vi "Close.vi"(8 "error in (no error)":errorcluster, 11 "IVI_Class in":refnum<class "IVI_Class.lvclass">) -> (0 "error out":errorcluster, 3 "IVI_Class out":refnum<class "IVI_Class.lvclass">)   [LabVIEW 2018, in "ScopePlugins.lvlib" / "IVI_Class.lvclass"]
doc: "Closes the session to the instrument."
uses:
  IVI_Class.lvclass
  C:/projects/ICDAS/NistPluggableModules/Scope/ScopePlugins/ScopePluginBaseClass/ScopePluginsBase.lvclass
  ScopePluginBaseClass/ScopePluginsBase.lvclass/ScopePluginsBase.ctl
  ScopePluginBaseClass/Accessors/Read Channels.vi
  ScopePluginBaseClass/Accessors/Write Channels.vi
  ScopePluginBaseClass/ScopePluginsBase.lvclass
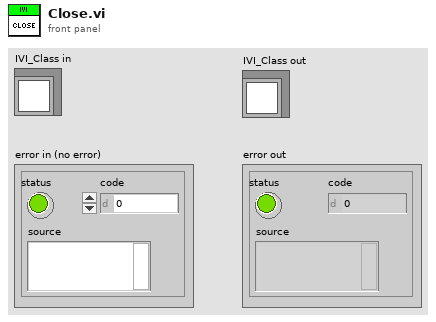
[diagram p1: front panel]
types:
  T1 = typedef "ScopePlugins.lvlib/ScopePluginsBase.lvclass/ChannelSetting(s).ctl" = cluster{"Number of Channels":i32, "Channel(s)":cluster{"Enabled":bool, "Instrument Handle":string, "Channel Name":string, "Maximum Input Frequency":dbl, "Verticle Settings":cluster{"Vertical Range":dbl, "Vertical Offset":dbl, "Probe Attenuation":dbl, "Vertical Coupling":i32}, "Connected":bool, "Input Impedance":dbl, "IO Type Instrument Handle":refnum<k15>}[]}
  T2 = cluster{"Enabled":bool, "Instrument Handle":string, "Channel Name":string, "Maximum Input Frequency":dbl, "Verticle Settings":cluster{"Vertical Range":dbl, "Vertical Offset":dbl, "Probe Attenuation":dbl, "Vertical Coupling":i32}, "Connected":bool, "Input Impedance":dbl, "IO Type Instrument Handle":refnum<k15>}[]
  T3 = cluster{"Enabled":bool, "Instrument Handle":string, "Channel Name":string, "Maximum Input Frequency":dbl, "Verticle Settings":cluster{"Vertical Range":dbl, "Vertical Offset":dbl, "Probe Attenuation":dbl, "Vertical Coupling":i32}, "Connected":bool, "Input Impedance":dbl, "IO Type Instrument Handle":refnum<k15>}
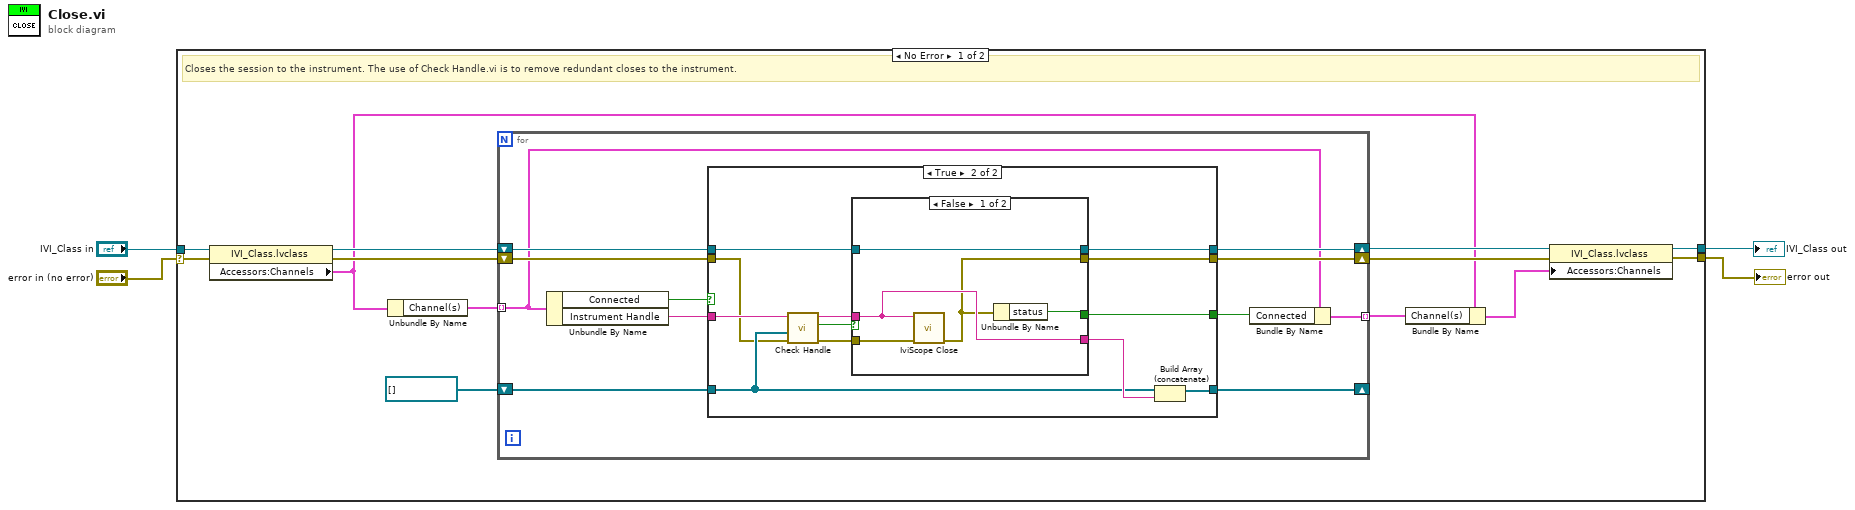
[diagram p0: block diagram]
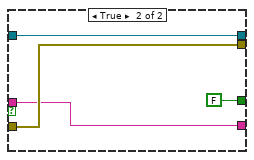
[diagram p3: hidden frame]
diagram:
  n1 = case shown="No Error" "error in (no error)" {
    selector: "error in (no error)" -> [w16 w54]
    tunnel: "IVI_Class in" -> [w17 w55]
    tunnel: [w11 w55] -> w4
    tunnel: [w9 w54] -> w2
    frame No Error {
      # "Closes the session to the instrument. The use of Check Handle.vi is to remove redundant closes to the instrument."
      n2 = property class="IVI_Class.lvclass"(reference=w17, error in=w16) -> (reference out=w15:refnum<class "IVI_Class.lvclass">, error out=w13:errorcluster, "Accessors:Channels"=w8:T1)
      n3 = Unbundle By Name(w8) -> ("Channel(s)"=w12:T2)
      n4 = for {
        shift-right: [w24] -> w14
        shift-left: w15 -> [w28]
        shift-right: [w25] -> w10
        shift-left: w13 -> [w27]
        tunnel: w12 -> [w19] mode=indexing
        tunnel: [w22] -> w7 mode=indexing
        shift-right: [w20] -> _
        shift-left: refnum<k15>[] [] -> [w21]
        n5 = Unbundle By Name(w19) -> ("Connected"=w18:bool, "Instrument Handle"=w26:string)
        n6 = case shown="True" w18 {
          selector: w18 -> [w30 _]
          tunnel: w28 -> [w32 w44]
          tunnel: w27 -> [w31 w34]
          tunnel: w26 -> [_ w36]
          tunnel: [w31 w43] -> w25
          tunnel: [w32 w42] -> w24
          tunnel: [w30 w41] -> w23
          tunnel: w21 -> [w29 w38]
          tunnel: [w29 w39] -> w20
          frame False {
          }
          frame True {
            n7 = call "Check Handle.vi"("error in (no error)"=w34, "Array"=w38, "Handle In"=w36) -> ("error out"=w33:errorcluster, "Duplicate Instrument?"=w37:bool, "Handle Out"=w35:string)  [unwired: 6 in]
            n8 = case shown="False" w37 {
              tunnel: w44 -> [w49 w53]
              tunnel: [w49 w53] -> w42
              tunnel: w33 -> [w48 w52]
              tunnel: [w46 w52] -> w43
              tunnel: [w45 FALSE] -> w41
              tunnel: [w47 w50] -> w40
              tunnel: w35 -> [w47 w50]
              frame False {
                n9 = call <vilib>:"IviScope Close.vi"("error in (no error)"=w48, "instrument handle"=w47) -> ("error out"=w46:errorcluster)  [unwired: 9 in]
                n10 = Unbundle By Name(w46) -> ("status"=w45:bool)
              }
              frame True {
              }
            }
            n11 = Build Array (concatenate)(w38, w40) -> (w39:refnum<k15>[])
          }
        }
        n12 = Bundle By Name(cluster=w19, "Connected"=w23) -> (w22:T3)
      }
      n13 = Bundle By Name(cluster=w8, "Channel(s)"=w7) -> (w6:T1)
      n14 = property class="IVI_Class.lvclass"(reference=w14, error in=w10, "Accessors:Channels"=w6) -> (reference out=w11:refnum<class "IVI_Class.lvclass">, error out=w9:errorcluster)
    }
    frame Error {
    }
  }
  "error out" <- w2
  "IVI_Class out" <- w4
